vi "Populate Run-Time Menu.vi"(8 "error in (no error)":errorcluster, 10 "Menu in":refnum<k9>, 11 "Execution UI In":refnum<class "Execution UI.lvclass">) -> (0 "error out":errorcluster, 3 "Execution UI Out":refnum<class "Execution UI.lvclass">)   [LabVIEW 2020, in "Execution UI.lvclass"]
uses:
  Execution UI.lvclass
  Execution UI.lvclass/Execution UI.ctl
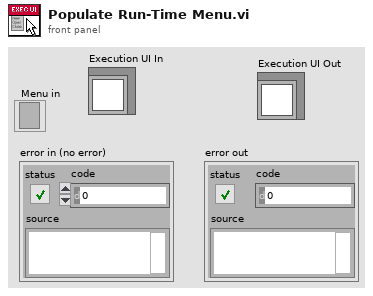
[diagram p1: front panel]
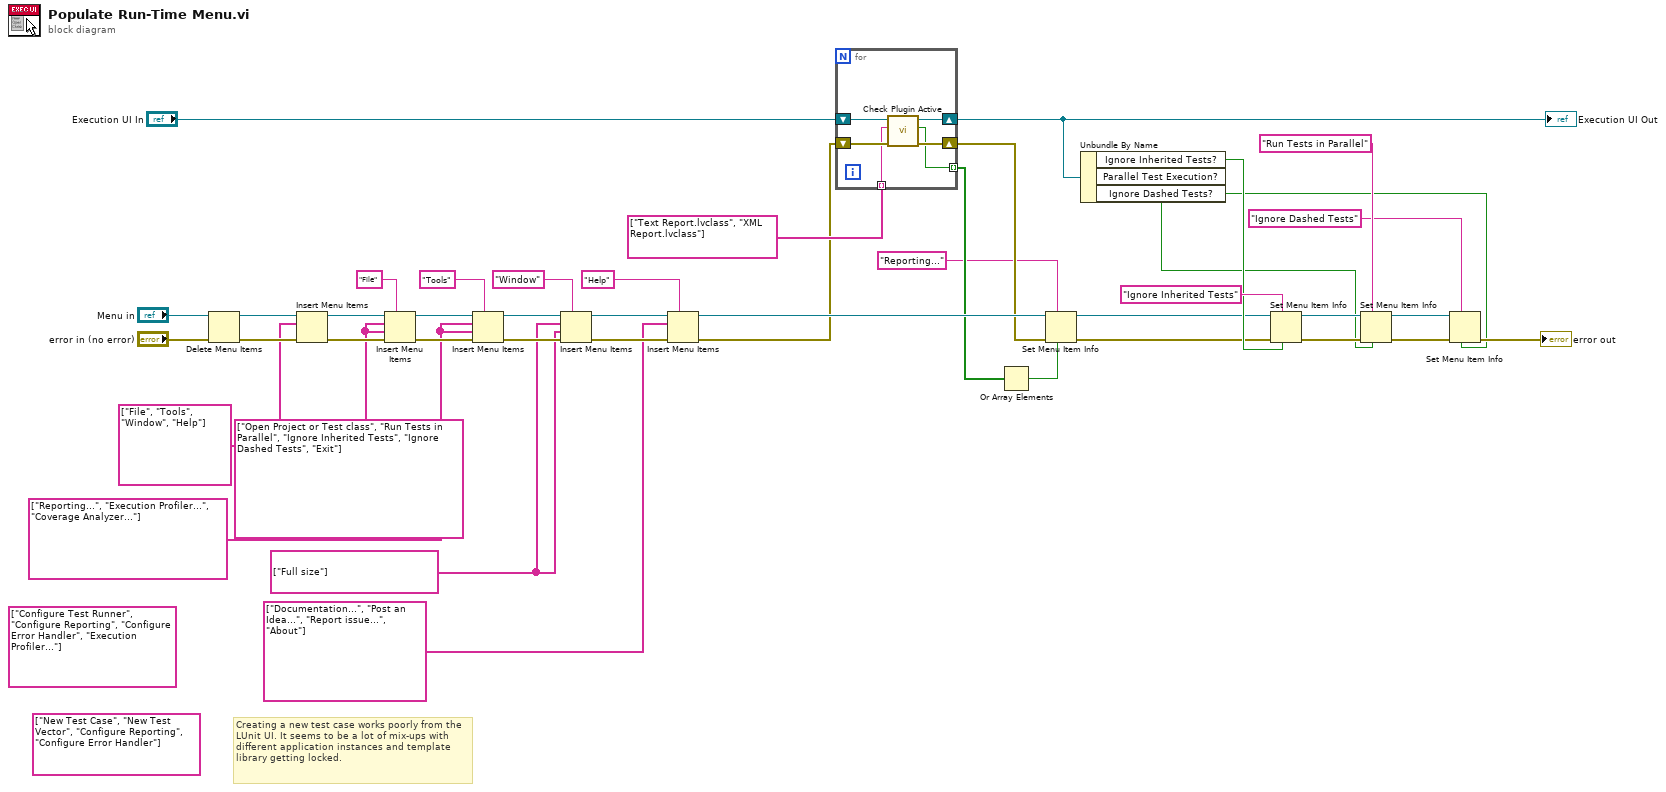
[diagram p0: block diagram]
diagram:
  (unwired) string[] ["Configure Test Runner", "Configure Reporting", "Configure Error Handler", "Execution Profiler..."] ("item names")
  (unwired) string[] ["New Test Case", "New Test Vector", "Configure Reporting", "Configure Error Handler"] ("item names")
  w24 = string[] ["Full size"] ("item names")
  w25 = string[] ["Reporting...", "Execution Profiler...", "Coverage Analyzer..."] ("item names")
  w22 = string[] ["Open Project or Test class", "Run Tests in Parallel", "Ignore Inherited Tests", "Ignore Dashed Tests", "Exit"] ("item names")
  # "Creating a new test case works poorly from the LUnit UI. It seems to be a lot of mix-ups with different application instances and template library getting locked."
  n1 = Delete Menu Items(6:"error in (no error)", 9:"Menu in") -> (0:w40:errorcluster, 3:w42:refnum<k9>)  [unwired: 2 in]
  n2 = Insert Menu Items(6:w40, 8:string[] ["File", "Tools", "Window", "Help"] ("item names"), 9:w42) -> (0:w37:errorcluster, 3:w38:refnum<k9>)  [unwired: 3 in, 1 out]
  n3 = Insert Menu Items(5:"File" ("menu tag"), 6:w37, 7:w22, 8:w22, 9:w38) -> (0:w33:errorcluster, 3:w32:refnum<k9>)  [unwired: 1 in, 1 out]
  n4 = Insert Menu Items(5:"Tools", 6:w33, 7:w25, 8:w25, 9:w32) -> (0:w34:errorcluster, 3:w31:refnum<k9>)  [unwired: 1 in, 1 out]
  n5 = Insert Menu Items(5:"Window", 6:w34, 7:w24, 8:w24, 9:w31) -> (0:w35:errorcluster, 3:w30:refnum<k9>)  [unwired: 1 in, 1 out]
  n6 = Insert Menu Items(5:"Help", 6:w35, 8:string[] ["Documentation...", "Post an Idea...", "Report issue...", "About"] ("item names"), 9:w30) -> (0:w9:errorcluster, 3:w15:refnum<k9>)  [unwired: 2 in, 1 out]
  n7 = for {
    shift-right: [w48] -> w12
    shift-left: "Execution UI In" -> [w49]
    shift-right: [w46] -> w8
    shift-left: w9 -> [w47]
    tunnel: string[] ["Text Report.lvclass", "XML Report.lvclass"] ("Plugin") -> [w45] mode=indexing
    tunnel: [w44] -> w10 mode=indexing
    n8 = call "Check Plugin Active.vi"("error in (no error)"=w47, "Plugin"=w45, "Execution UI in"=w49) -> ("error out"=w46:errorcluster, "Active?"=w44:bool, "Execution UI out"=w48:refnum<class "Execution UI.lvclass">)  [unwired: 6 in]
  }
  "Execution UI Out" <- w12
  n9 = Or Array Elements(Boolean array=w10) -> (logical OR=w7:bool)
  n10 = Set Menu Item Info(6:w7, 7:"Reporting...", 8:w8, 11:w15) -> (0:w16:errorcluster, 3:w14:refnum<k9>)  [unwired: 3 in]
  n11 = Unbundle By Name(w12) -> ("Ignore Inherited Tests?"=w21:bool, "Parallel Test Execution?"=w17:bool, "Ignore Dashed Tests?"=w1:bool)
  n12 = Set Menu Item Info(6:w21, 7:"Ignore Inherited Tests", 8:w16, 11:w14) -> (0:w19:errorcluster, 3:w18:refnum<k9>)  [unwired: 3 in]
  n13 = Set Menu Item Info(6:w17, 7:"Run Tests in Parallel", 8:w19, 11:w18) -> (0:w4:errorcluster, 3:w5:refnum<k9>)  [unwired: 3 in]
  n14 = Set Menu Item Info(6:w1, 7:"Ignore Dashed Tests", 8:w4, 11:w5) -> (0:→"error out":errorcluster)  [unwired: 3 in, 1 out]
